vi "Write Index.vi"(8 "error in (no error)":errorcluster, 10 "Index":i32, 11 "abs_Composite in":refnum<class "abs_Composite.lvclass">) -> (0 "error out":errorcluster, 3 "abs_Composite out":refnum<class "abs_Composite.lvclass">)   [LabVIEW 2021, in "BT.lvlib" / "abs_Composite.lvclass"]
uses:
  abs_Composite.lvclass
  abs_Composite.lvclass/abs_Composite.ctl
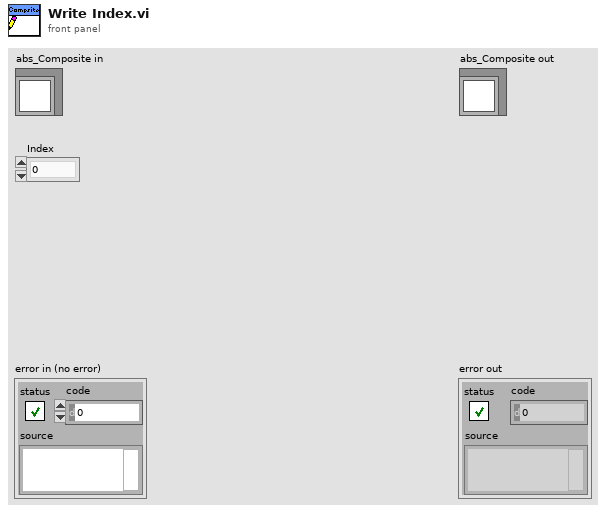
[diagram p1: front panel]
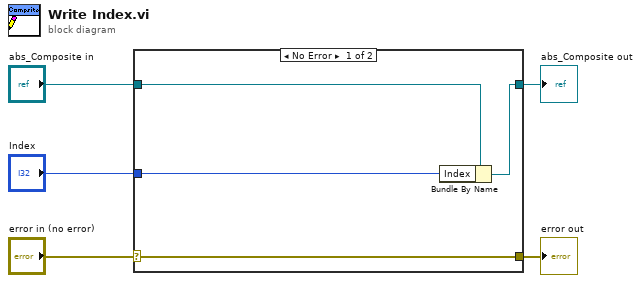
[diagram p0: block diagram]
diagram:
  n1 = case shown="No Error" "error in (no error)" {
    selector: "error in (no error)" -> [w9 w10]
    tunnel: [w9 w10] -> w4
    tunnel: [w7 w11] -> w2
    tunnel: "abs_Composite in" -> [w8 w11]
    tunnel: "Index" -> [w6 _]
    frame No Error {
      n2 = Bundle By Name(cluster=w8, "Index"=w6) -> (w7:refnum<class "abs_Composite.lvclass">)
    }
    frame Error {
    }
  }
  "error out" <- w4
  "abs_Composite out" <- w2
